vi "Destroy.vi"(8 "Error In":errorcluster, 11 "Animation In":refnum<class "Animation.lvclass">) -> (0 "Error Out":errorcluster)   [LabVIEW 2021, in "Animation.lvclass"]
uses:
  Animation.lvclass
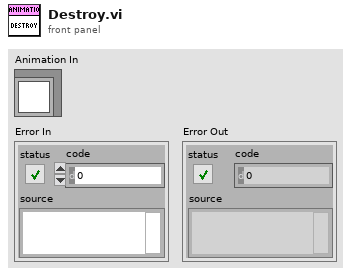
[diagram p1: front panel]
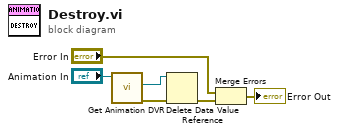
[diagram p0: block diagram]
diagram:
  n1 = call "Get Animation DVR.vi"("Animation In"="Animation In") -> ("Error Out"=w5:errorcluster, "DVR"=w4:refnum<data-value>)  [unwired: 8 in, 1 out]
  n2 = Delete Data Value Reference(data value reference=w4, error in=w5) -> (error out=w2:errorcluster)  [unwired: 1 out]
  n3 = Merge Errors("Error In", w2) -> (→"Error Out":errorcluster)
